vi "LM Two Asymmetric Gaussians and gradient.vi"(3 "output control":T1, 4 "data":variant, 5 "X":dbl[](array[numeric]), 6 "a":dbl[](array[numeric])) -> (0 "error out":errorcluster, 1 "f'(X,a)":dbl[][](array[numeric]), 2 "f(X,a)":dbl[](array[numeric]))   [LabVIEW 2021, in "Fits.lvlib"]
doc: "This template is the starting point for creating a model function to be passed to the Nonlinear Curve Fit.vi."
uses:
  Fits.lvlib
  <vilib>/gmath/NumericalOptimization/LM_output select.ctl
  D-Only Fixed Parameters.ctl
  <vilib>/gmath/NI_Gmath.lvlib
panel:
  # "Parameters:\n\namplitude 1: A1\ncenter 1: t1\nSDV 1-: s1-\nSDV 1+: s1+\nAmplitude 2: A2\ncenter 2: t2\nSDV 2-: s2-\nSDV 2+: s2+"
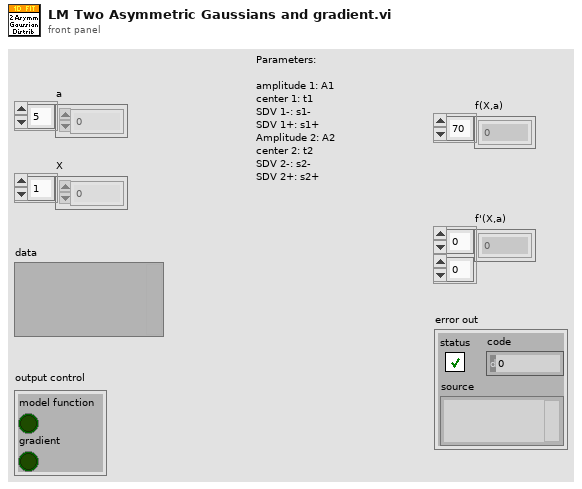
[diagram p1: front panel]
types:
  T1 = typedef "NI_Gmath.lvlib/LM_output select.ctl" = cluster{"model function":bool, "gradient":bool}
  T2 = typedef "Fits.lvlib/D-Only Fixed Parameters.ctl" = cluster{"Fix D-only Peak Location":bool, "Peak Location":dbl, "Fix D-only Peak FWHM":bool, "Peak FWHM":dbl}
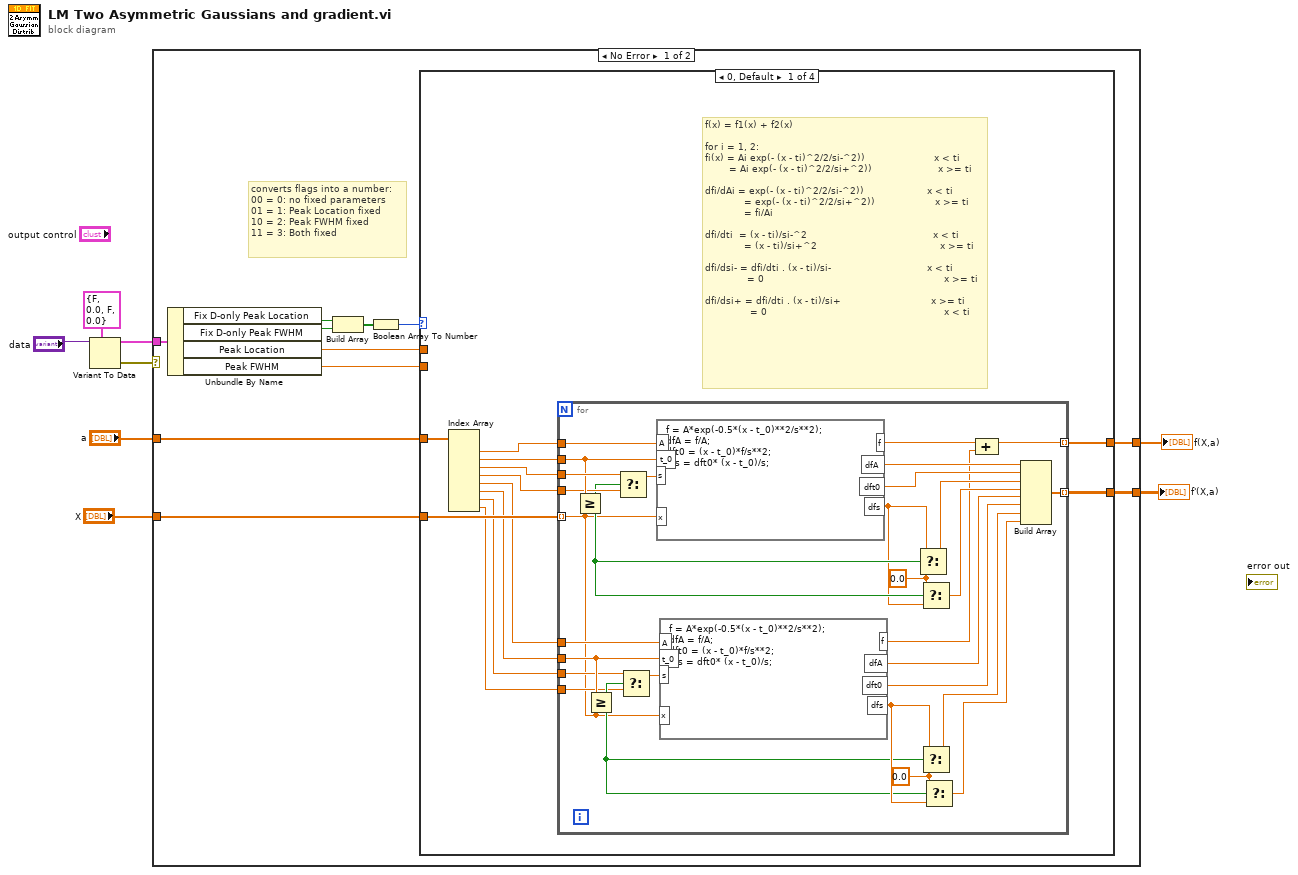
[diagram p0: block diagram]
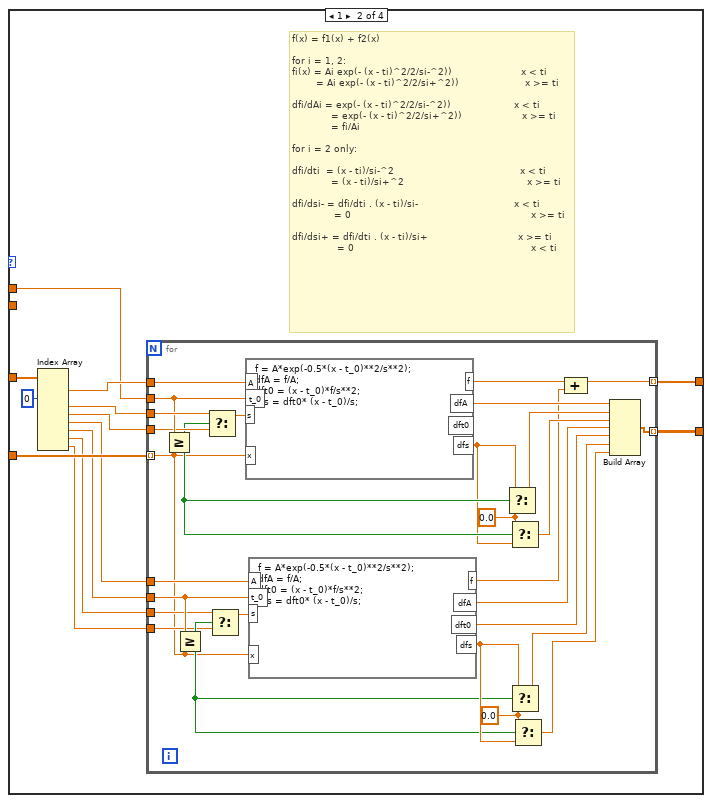
[diagram p2: hidden frame]
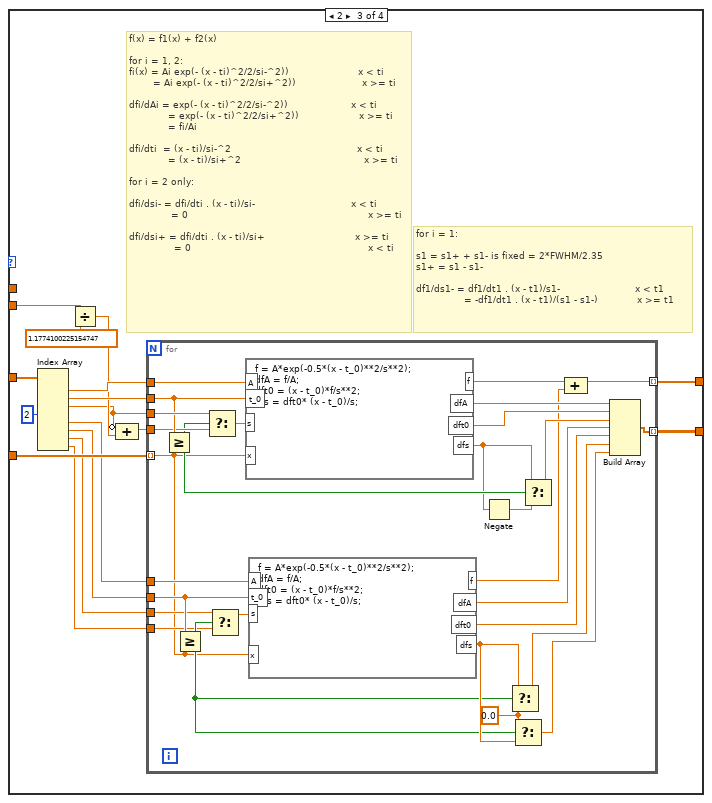
[diagram p3: hidden frame]
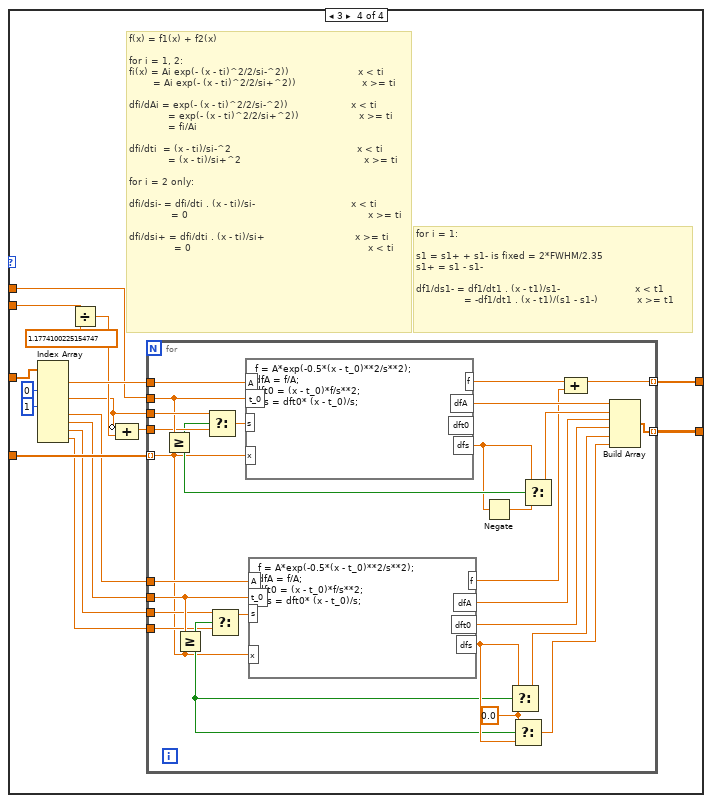
[diagram p4: hidden frame]
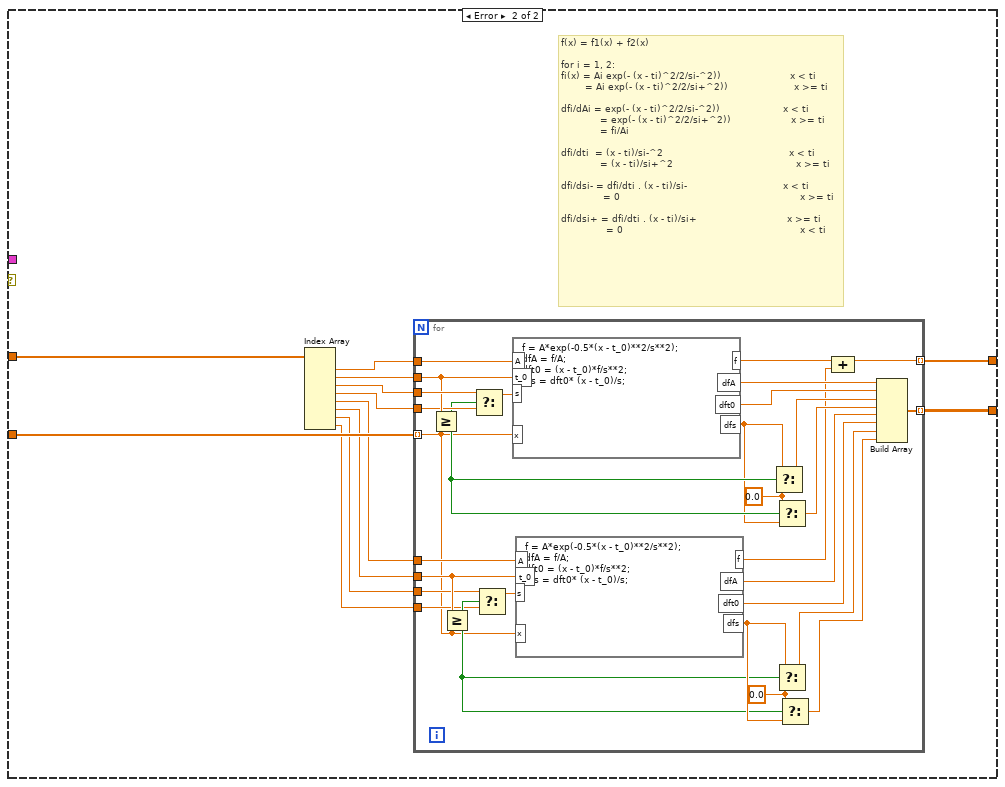
[diagram p5: hidden frame]
diagram:
  n1 = Variant To Data(type=T2 {"Fix D-only Peak Location"=FALSE, "Peak Location"=0.0, "Fix D-only Peak FWHM"=FALSE, "Peak FWHM"=0.0} ("Fixed Parameters"), Variant="data") -> (data=w1:T2, error out=w2:errorcluster)  [unwired: 1 in]
  n2 = case shown="No Error" w2 {
    tunnel: "a" -> [w19 w201]
    tunnel: "X" -> [w18 w196]
    tunnel: [w17 w191] -> w6
    tunnel: [w16 w190] -> w5
    tunnel: w1 -> [w12 _]
    frame No Error {
      # "converts flags into a number:\n00 = 0: no fixed parameters\n01 = 1: Peak Location fixed\n10 = 2: Peak FWHM fixed\n11 = 3: Both fixed"
      n3 = Unbundle By Name(w12) -> ("Fix D-only Peak Location"=w15:bool, "Fix D-only Peak FWHM"=w14:bool, "Peak Location"=w10:dbl, "Peak FWHM"=w9:dbl)
      n4 = Build Array(w15, w14) -> (w13:bool[])
      n5 = Boolean Array To Number(Boolean array=w13) -> (number=w11:u32)
      n6 = case shown="0, Default" w11 {
        tunnel: w19 -> [w31 w73 w117 w162]
        tunnel: w18 -> [w26 w69 w114 w160]
        tunnel: [w21 w64 w109 w155] -> w17
        tunnel: [w20 w63 w108 w154] -> w16
        tunnel: w10 -> [_ w62 _ w147]
        tunnel: w9 -> [_ _ w107 w153]
        frame 0, Default {
          # "f(x) = f1(x) + f2(x)\n\nfor i = 1, 2: \nfi(x) = Ai exp(- (x - ti)^2/2/si-^2))                       x < ti\n        = Ai exp(- (x - ti)^2/2/si+^2))                      x >= ti\n\ndfi/dAi = exp(- (x - ti)^2/2/si-^2))                     x < ti\n             = exp(- (x - ti)^2/2/si+^2))                    x >= ti\n             = fi/Ai\n\ndfi/dti  = (x - ti)/si-^2                                          x < ti\n             = (x - ti)/si+^2                                         x >= ti\n\ndfi/dsi- = dfi/dti . (x - ti)/si-                                x < ti\n              = 0                                                            x >= ti\n\ndfi/dsi+ = dfi/dti . (x - ti)/si+                              x >= ti\n               = 0                                                           x < ti"
          n7 = Index Array(array=w31) -> (element #1=w30:dbl, element #2=w29:dbl, element #3=w28:dbl, element #4=w27:dbl, element #5=w25:dbl, element #6=w24:dbl, element #7=w23:dbl, element #8=w22:dbl)  [unwired: 8 in]
          n8 = for {
            tunnel: w30 -> [w60]
            tunnel: w29 -> [w57]
            tunnel: w28 -> [w59]
            tunnel: w27 -> [w56]
            tunnel: w26 -> [w38] mode=indexing
            tunnel: [w37] -> w21 mode=indexing
            tunnel: [w47] -> w20 mode=indexing
            tunnel: w25 -> [w42]
            tunnel: w24 -> [w41]
            tunnel: w23 -> [w40]
            tunnel: w22 -> [w39]
            w45 = 0.0 ("f")
            w54 = 0.0 ("f")
            n9 = Greater Or Equal?(x=w57, y=w38) -> (x >= y?=w55:bool)
            n10 = Greater Or Equal?(x=w41, y=w38) -> (x >= y?=w44:bool)
            n11 = Select(t=w59, s=w55, f=w56) -> (s? t:f=w58:dbl)
            n12 = Select(t=w40, s=w44, f=w39) -> (s? t:f=w43:dbl)
            n13 = formula code="f = A*exp(-0.5*(x - t_0)**2/s**2);\ndfA = f/A;\ndft0 = (x - t_0)*f/s**2;\ndfs = dft0* (x - t_0)/s;"("A"=w60, "t_0"=w57, "s"=w58, "x"=w38) -> ("f"=w51:dbl, "dfA"=w52:dbl, "dft0"=w50:dbl, "dfs"=w53:dbl)
            n14 = formula code="f = A*exp(-0.5*(x - t_0)**2/s**2);\ndfA = f/A;\ndft0 = (x - t_0)*f/s**2;\ndfs = dft0* (x - t_0)/s;"("A"=w42, "t_0"=w41, "s"=w43, "x"=w38) -> ("f"=w36:dbl, "dfA"=w35:dbl, "dft0"=w34:dbl, "dfs"=w46:dbl)
            n15 = Select(t=w53, s=w55, f=w54) -> (s? t:f=w49:dbl)
            n16 = Select(t=w54, s=w55, f=w53) -> (s? t:f=w48:dbl)
            n17 = Select(t=w46, s=w44, f=w45) -> (s? t:f=w33:dbl)
            n18 = Select(t=w45, s=w44, f=w46) -> (s? t:f=w32:dbl)
            n19 = Compound Arithmetic op=ADD(w51, w36) -> (w37:dbl)
            n20 = Build Array(w52, w50, w49, w48, w35, w34, w33, w32) -> (w47:dbl[])
          }
        }
        frame 1 {
          # "f(x) = f1(x) + f2(x)\n\nfor i = 1, 2: \nfi(x) = Ai exp(- (x - ti)^2/2/si-^2))                       x < ti\n        = Ai exp(- (x - ti)^2/2/si+^2))                      x >= ti\n\ndfi/dAi = exp(- (x - ti)^2/2/si-^2))                     x < ti\n             = exp(- (x - ti)^2/2/si+^2))                    x >= ti\n             = fi/Ai\n\nfor i = 2 only: \n\ndfi/dti  = (x - ti)/si-^2                                          x < ti\n             = (x - ti)/si+^2                                         x >= ti\n\ndfi/dsi- = dfi/dti . (x - ti)/si-                                x < ti\n              = 0                                                            x >= ti\n\ndfi/dsi+ = dfi/dti . (x - ti)/si+                              x >= ti\n               = 0                                                           x < ti"
          n21 = Index Array(array=w73, index #2=0 ("index")) -> (element #1=w72:dbl, element #3=w71:dbl, element #4=w70:dbl, element #5=w68:dbl, element #6=w67:dbl, element #7=w66:dbl, element #8=w65:dbl)  [unwired: 7 in, 1 out]
          n22 = for {
            tunnel: w72 -> [w101]
            tunnel: w62 -> [w98]
            tunnel: w71 -> [w100]
            tunnel: w70 -> [w97]
            tunnel: w69 -> [w80] mode=indexing
            tunnel: [w79] -> w64 mode=indexing
            tunnel: [w89] -> w63 mode=indexing
            tunnel: w68 -> [w84]
            tunnel: w67 -> [w83]
            tunnel: w66 -> [w82]
            tunnel: w65 -> [w81]
            w87 = 0.0 ("f")
            w95 = 0.0 ("f")
            n23 = Greater Or Equal?(x=w98, y=w80) -> (x >= y?=w96:bool)
            n24 = Greater Or Equal?(x=w83, y=w80) -> (x >= y?=w86:bool)
            n25 = Select(t=w100, s=w96, f=w97) -> (s? t:f=w99:dbl)
            n26 = Select(t=w82, s=w86, f=w81) -> (s? t:f=w85:dbl)
            n27 = formula code="f = A*exp(-0.5*(x - t_0)**2/s**2);\ndfA = f/A;\ndft0 = (x - t_0)*f/s**2;\ndfs = dft0* (x - t_0)/s;"("A"=w101, "t_0"=w98, "s"=w99, "x"=w80) -> ("f"=w92:dbl, "dfA"=w93:dbl, "dfs"=w94:dbl)  [unwired: 1 out]
            n28 = formula code="f = A*exp(-0.5*(x - t_0)**2/s**2);\ndfA = f/A;\ndft0 = (x - t_0)*f/s**2;\ndfs = dft0* (x - t_0)/s;"("A"=w84, "t_0"=w83, "s"=w85, "x"=w80) -> ("f"=w78:dbl, "dfA"=w77:dbl, "dft0"=w76:dbl, "dfs"=w88:dbl)
            n29 = Select(t=w94, s=w96, f=w95) -> (s? t:f=w91:dbl)
            n30 = Select(t=w95, s=w96, f=w94) -> (s? t:f=w90:dbl)
            n31 = Select(t=w88, s=w86, f=w87) -> (s? t:f=w75:dbl)
            n32 = Select(t=w87, s=w86, f=w88) -> (s? t:f=w74:dbl)
            n33 = Compound Arithmetic op=ADD(w92, w78) -> (w79:dbl)
            n34 = Build Array(w93, w91, w90, w77, w76, w75, w74) -> (w89:dbl[])
          }
        }
        frame 2 {
          # "for i = 1: \n\ns1 = s1+ + s1- is fixed = 2*FWHM/2.35\ns1+ = s1 - s1-\n\ndf1/ds1- = df1/dt1 . (x - t1)/s1-                         x < t1\n                = -df1/dt1 . (x - t1)/(s1 - s1-)             x >= t1"
          # "f(x) = f1(x) + f2(x)\n\nfor i = 1, 2: \nfi(x) = Ai exp(- (x - ti)^2/2/si-^2))                       x < ti\n        = Ai exp(- (x - ti)^2/2/si+^2))                      x >= ti\n\ndfi/dAi = exp(- (x - ti)^2/2/si-^2))                     x < ti\n             = exp(- (x - ti)^2/2/si+^2))                    x >= ti\n             = fi/Ai\n\ndfi/dti  = (x - ti)/si-^2                                          x < ti\n             = (x - ti)/si+^2                                         x >= ti\n\nfor i = 2 only: \n\ndfi/dsi- = dfi/dti . (x - ti)/si-                                x < ti\n              = 0                                                            x >= ti\n\ndfi/dsi+ = dfi/dti . (x - ti)/si+                              x >= ti\n               = 0                                                           x < ti"
          n35 = Index Array(array=w117, index #4=2 ("index")) -> (element #1=w116:dbl, element #2=w115:dbl, element #3=w103:dbl, element #5=w113:dbl, element #6=w112:dbl, element #7=w111:dbl, element #8=w110:dbl)  [unwired: 7 in, 1 out]
          n36 = Divide(x=w107, y=1.1774100225154747) -> (x/y=w104:dbl)
          n37 = Compound Arithmetic op=ADD(invert w103, w104) -> (w102:dbl)
          n38 = for {
            tunnel: w116 -> [w145]
            tunnel: w115 -> [w142]
            tunnel: w103 -> [w144]
            tunnel: w102 -> [w141]
            tunnel: w114 -> [w126] mode=indexing
            tunnel: [w125] -> w109 mode=indexing
            tunnel: [w135] -> w108 mode=indexing
            tunnel: w113 -> [w130]
            tunnel: w112 -> [w129]
            tunnel: w111 -> [w128]
            tunnel: w110 -> [w127]
            w133 = 0.0 ("f")
            n39 = Greater Or Equal?(x=w142, y=w126) -> (x >= y?=w140:bool)
            n40 = Greater Or Equal?(x=w129, y=w126) -> (x >= y?=w132:bool)
            n41 = Select(t=w144, s=w140, f=w141) -> (s? t:f=w143:dbl)
            n42 = Select(t=w128, s=w132, f=w127) -> (s? t:f=w131:dbl)
            n43 = formula code="f = A*exp(-0.5*(x - t_0)**2/s**2);\ndfA = f/A;\ndft0 = (x - t_0)*f/s**2;\ndfs = dft0* (x - t_0)/s;"("A"=w145, "t_0"=w142, "s"=w143, "x"=w126) -> ("f"=w138:dbl, "dfA"=w139:dbl, "dft0"=w137:dbl, "dfs"=w119:dbl)
            n44 = formula code="f = A*exp(-0.5*(x - t_0)**2/s**2);\ndfA = f/A;\ndft0 = (x - t_0)*f/s**2;\ndfs = dft0* (x - t_0)/s;"("A"=w130, "t_0"=w129, "s"=w131, "x"=w126) -> ("f"=w124:dbl, "dfA"=w123:dbl, "dft0"=w122:dbl, "dfs"=w134:dbl)
            n45 = Negate(x=w119) -> (-x=w118:dbl)
            n46 = Select(t=w134, s=w132, f=w133) -> (s? t:f=w121:dbl)
            n47 = Select(t=w133, s=w132, f=w134) -> (s? t:f=w120:dbl)
            n48 = Select(t=w119, s=w140, f=w118) -> (s? t:f=w136:dbl)
            n49 = Compound Arithmetic op=ADD(w138, w124) -> (w125:dbl)
            n50 = Build Array(w139, w137, w136, w123, w122, w121, w120) -> (w135:dbl[])
          }
        }
        frame 3 {
          # "for i = 1: \n\ns1 = s1+ + s1- is fixed = 2*FWHM/2.35\ns1+ = s1 - s1-\n\ndf1/ds1- = df1/dt1 . (x - t1)/s1-                         x < t1\n                = -df1/dt1 . (x - t1)/(s1 - s1-)             x >= t1"
          # "f(x) = f1(x) + f2(x)\n\nfor i = 1, 2: \nfi(x) = Ai exp(- (x - ti)^2/2/si-^2))                       x < ti\n        = Ai exp(- (x - ti)^2/2/si+^2))                      x >= ti\n\ndfi/dAi = exp(- (x - ti)^2/2/si-^2))                     x < ti\n             = exp(- (x - ti)^2/2/si+^2))                    x >= ti\n             = fi/Ai\n\ndfi/dti  = (x - ti)/si-^2                                          x < ti\n             = (x - ti)/si+^2                                         x >= ti\n\nfor i = 2 only: \n\ndfi/dsi- = dfi/dti . (x - ti)/si-                                x < ti\n              = 0                                                            x >= ti\n\ndfi/dsi+ = dfi/dti . (x - ti)/si+                              x >= ti\n               = 0                                                           x < ti"
          n51 = Index Array(array=w162, index #2=0 ("index"), index #4=1 ("index")) -> (element #1=w161:dbl, element #3=w149:dbl, element #5=w159:dbl, element #6=w158:dbl, element #7=w157:dbl, element #8=w156:dbl)  [unwired: 6 in, 2 out]
          n52 = Divide(x=w153, y=1.1774100225154747) -> (x/y=w150:dbl)
          n53 = Compound Arithmetic op=ADD(invert w149, w150) -> (w148:dbl)
          n54 = for {
            tunnel: w161 -> [w189]
            tunnel: w147 -> [w186]
            tunnel: w149 -> [w188]
            tunnel: w148 -> [w185]
            tunnel: w160 -> [w171] mode=indexing
            tunnel: [w170] -> w155 mode=indexing
            tunnel: [w180] -> w154 mode=indexing
            tunnel: w159 -> [w175]
            tunnel: w158 -> [w174]
            tunnel: w157 -> [w173]
            tunnel: w156 -> [w172]
            w178 = 0.0 ("f")
            n55 = Greater Or Equal?(x=w186, y=w171) -> (x >= y?=w184:bool)
            n56 = Greater Or Equal?(x=w174, y=w171) -> (x >= y?=w177:bool)
            n57 = Select(t=w188, s=w184, f=w185) -> (s? t:f=w187:dbl)
            n58 = Select(t=w173, s=w177, f=w172) -> (s? t:f=w176:dbl)
            n59 = formula code="f = A*exp(-0.5*(x - t_0)**2/s**2);\ndfA = f/A;\ndft0 = (x - t_0)*f/s**2;\ndfs = dft0* (x - t_0)/s;"("A"=w189, "t_0"=w186, "s"=w187, "x"=w171) -> ("f"=w182:dbl, "dfA"=w183:dbl, "dfs"=w164:dbl)  [unwired: 1 out]
            n60 = formula code="f = A*exp(-0.5*(x - t_0)**2/s**2);\ndfA = f/A;\ndft0 = (x - t_0)*f/s**2;\ndfs = dft0* (x - t_0)/s;"("A"=w175, "t_0"=w174, "s"=w176, "x"=w171) -> ("f"=w169:dbl, "dfA"=w168:dbl, "dft0"=w167:dbl, "dfs"=w179:dbl)
            n61 = Negate(x=w164) -> (-x=w163:dbl)
            n62 = Select(t=w179, s=w177, f=w178) -> (s? t:f=w166:dbl)
            n63 = Select(t=w178, s=w177, f=w179) -> (s? t:f=w165:dbl)
            n64 = Select(t=w164, s=w184, f=w163) -> (s? t:f=w181:dbl)
            n65 = Compound Arithmetic op=ADD(w182, w169) -> (w170:dbl)
            n66 = Build Array(w183, w181, w168, w167, w166, w165) -> (w180:dbl[])
          }
        }
      }
    }
    frame Error {
      # "f(x) = f1(x) + f2(x)\n\nfor i = 1, 2: \nfi(x) = Ai exp(- (x - ti)^2/2/si-^2))                       x < ti\n        = Ai exp(- (x - ti)^2/2/si+^2))                      x >= ti\n\ndfi/dAi = exp(- (x - ti)^2/2/si-^2))                     x < ti\n             = exp(- (x - ti)^2/2/si+^2))                    x >= ti\n             = fi/Ai\n\ndfi/dti  = (x - ti)/si-^2                                          x < ti\n             = (x - ti)/si+^2                                         x >= ti\n\ndfi/dsi- = dfi/dti . (x - ti)/si-                                x < ti\n              = 0                                                            x >= ti\n\ndfi/dsi+ = dfi/dti . (x - ti)/si+                              x >= ti\n               = 0                                                           x < ti"
      n67 = Index Array(array=w201) -> (element #1=w200:dbl, element #2=w199:dbl, element #3=w198:dbl, element #4=w197:dbl, element #5=w195:dbl, element #6=w194:dbl, element #7=w193:dbl, element #8=w192:dbl)  [unwired: 8 in]
      n68 = for {
        tunnel: w200 -> [w230]
        tunnel: w199 -> [w227]
        tunnel: w198 -> [w229]
        tunnel: w197 -> [w226]
        tunnel: w196 -> [w208] mode=indexing
        tunnel: [w207] -> w191 mode=indexing
        tunnel: [w217] -> w190 mode=indexing
        tunnel: w195 -> [w212]
        tunnel: w194 -> [w211]
        tunnel: w193 -> [w210]
        tunnel: w192 -> [w209]
        w215 = 0.0 ("f")
        w224 = 0.0 ("f")
        n69 = Greater Or Equal?(x=w227, y=w208) -> (x >= y?=w225:bool)
        n70 = Greater Or Equal?(x=w211, y=w208) -> (x >= y?=w214:bool)
        n71 = Select(t=w229, s=w225, f=w226) -> (s? t:f=w228:dbl)
        n72 = Select(t=w210, s=w214, f=w209) -> (s? t:f=w213:dbl)
        n73 = formula code="f = A*exp(-0.5*(x - t_0)**2/s**2);\ndfA = f/A;\ndft0 = (x - t_0)*f/s**2;\ndfs = dft0* (x - t_0)/s;"("A"=w230, "t_0"=w227, "s"=w228, "x"=w208) -> ("f"=w221:dbl, "dfA"=w222:dbl, "dft0"=w220:dbl, "dfs"=w223:dbl)
        n74 = formula code="f = A*exp(-0.5*(x - t_0)**2/s**2);\ndfA = f/A;\ndft0 = (x - t_0)*f/s**2;\ndfs = dft0* (x - t_0)/s;"("A"=w212, "t_0"=w211, "s"=w213, "x"=w208) -> ("f"=w206:dbl, "dfA"=w205:dbl, "dft0"=w204:dbl, "dfs"=w216:dbl)
        n75 = Select(t=w223, s=w225, f=w224) -> (s? t:f=w219:dbl)
        n76 = Select(t=w224, s=w225, f=w223) -> (s? t:f=w218:dbl)
        n77 = Select(t=w216, s=w214, f=w215) -> (s? t:f=w203:dbl)
        n78 = Select(t=w215, s=w214, f=w216) -> (s? t:f=w202:dbl)
        n79 = Compound Arithmetic op=ADD(w221, w206) -> (w207:dbl)
        n80 = Build Array(w222, w220, w219, w218, w205, w204, w203, w202) -> (w217:dbl[])
      }
    }
  }
  "f(X,a)" <- w6
  "f'(X,a)" <- w5
